vi "TDMS Reader.vi"() -> ()   [LabVIEW 2010]
panel:
  out "테스트 시간":timestamp=timestamp(-9593226000 s since 1904-01-01)
  out "테스트 수행자":string
  out "채널 데이터":waveform(dbl)(graph)
  in  "데이터 세트":string(combo)="시간 데이터"
  in  "시리얼 번호":string
  in  "TDMS 파일 경로":path=path "D:/Exercises/LabVIEW Core 2/TDMS Logger/Test Data.tdms" caption="TDMS파일 경로"
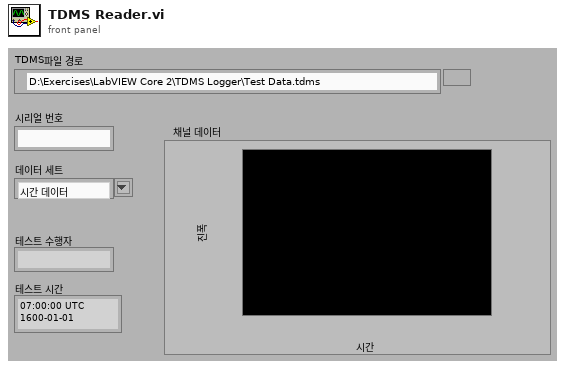
[diagram p1: front panel]
types:
  T1 = enum16{"open", "open or create", "create or replace", "create", "open (read-only)"}
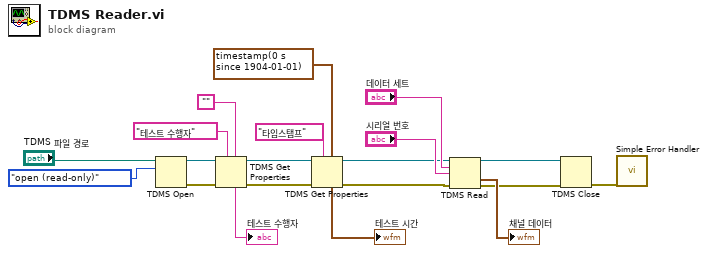
[diagram p0: block diagram]
diagram:
  n1 = TDMS Open(10:T1."open (read-only)" ("operation (0:open)"), 11:"TDMS 파일 경로") -> (0:w12:errorcluster, 3:w13:refnum<k34>)  [unwired: 4 in]
  n2 = TDMS Get Properties(5:"", 7:"테스트 수행자" ("property name"), 8:w12, 11:w13) -> (0:w9:errorcluster, 3:w11:refnum<k34>, 4:→"테스트 수행자":string)  [unwired: 5 out]
  n3 = TDMS Get Properties(5:timestamp(0 s since 1904-01-01), 7:"타임스탬프" ("property name"), 8:w9, 11:w11) -> (0:w8:errorcluster, 3:w10:refnum<k34>, 4:→"테스트 시간":timestamp)  [unwired: 5 out]
  n4 = TDMS Read(0:w10, 5:"데이터 세트", 7:"시리얼 번호", 11:w8) -> (4:w16:refnum<k34>, 10:→"채널 데이터":waveform(dbl), 15:w1:errorcluster)  [unwired: 3 in, 3 out]
  n5 = TDMS Close(8:w1, 11:w16) -> (0:w14:errorcluster)  [unwired: 1 out]
  n6 = call <vilib>:"Simple Error Handler.vi"("error in (no error)"=w14) -> ()  [unwired: 1 in, 8 out]
